vi "MCL Write Value.vi"(8 "error in (no error)":errorcluster, 10 "Value":i32[](array[numeric]), 11 "MCL Ref (generic)":refnum<vi>) -> (0 "error out":errorcluster, 3 "MCL Ref (generic)":refnum<vi>)   [LabVIEW 2020, in "BetterDragAndDrop.lvlib" / "BetterMultiListboxHandle.lvclass"]
uses:
  BetterMultiListboxHandle.lvclass
  <vilib>/Utility/error.llb/Error Cluster From Error Code.vi
  <vilib>/ErrorRing/Error Ring.xnode
  BetterMultiListboxHandle.lvclass/BetterMultiListboxHandle.ctl
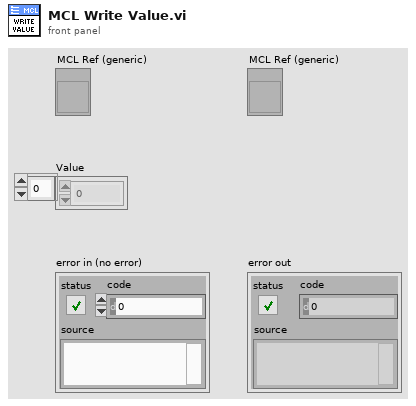
[diagram p1: front panel]
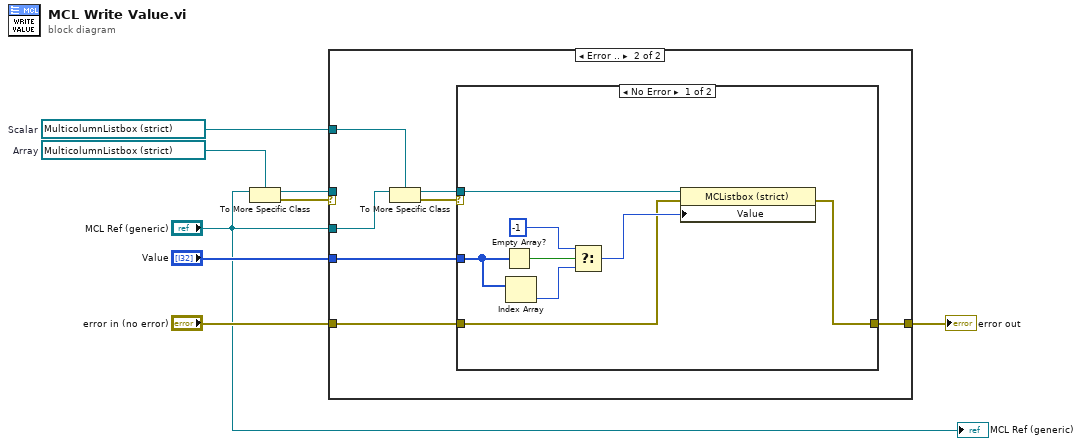
[diagram p0: block diagram]
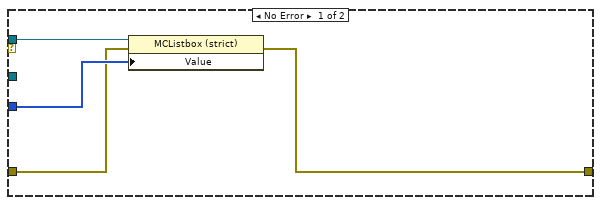
[diagram p2: hidden frame]
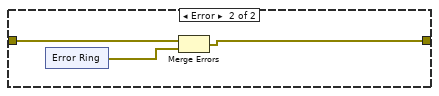
[diagram p3: hidden frame]
diagram:
  w8 = refnum<vi> refnum  # Array
  w5 = refnum<vi> refnum  # Scalar
  n1 = To More Specific Class(target class=w8, reference="MCL Ref (generic)") -> (specific class reference=w6:refnum<vi>, error out=w7:errorcluster)  [unwired: 1 in]
  n2 = case shown="Error .." w7 {
    tunnel: w6 -> [w12 _]
    tunnel: "MCL Ref (generic)" -> [_ w19]
    tunnel: w5 -> [_ w18]
    tunnel: "error in (no error)" -> [w10 w15]
    tunnel: [w9 w14] -> w3
    tunnel: "Value" -> [w11 w13]
    frame No Error {
      n3 = property class="MCListbox (strict)"(reference=w12, error in=w10, "Value"=w11) -> (error out=w9:errorcluster)  [unwired: 1 out]
    }
    frame Error {
      n4 = To More Specific Class(target class=w18, reference=w19) -> (specific class reference=w16:refnum<vi>, error out=w17:errorcluster)  [unwired: 1 in]
      n5 = case shown="No Error" w17 {
        tunnel: w16 -> [w27 _]
        tunnel: w15 -> [w21 w29]
        tunnel: [w20 w28] -> w14
        tunnel: w13 -> [w25 _]
        frame No Error {
          n6 = Empty Array?(array=w25) -> (empty?=w26:bool)
          n7 = Index Array(array=w25) -> (element=w24:i32)  [unwired: 1 in]
          n8 = Select(t=-1, s=w26, f=w24) -> (s? t:f=w22:i32)
          n9 = property class="MCListbox (strict)"(reference=w27, error in=w21, "Value"=w22) -> (error out=w20:errorcluster)  [unwired: 1 out]
        }
        frame Error {
          n10 = xnode "Error Ring"() -> ("error out"=w30:errorcluster)
          n11 = Merge Errors(w29, w30) -> (w28:errorcluster)
        }
      }
    }
  }
  "error out" <- w3
  "MCL Ref (generic)" <- "MCL Ref (generic)"
